vi "Update Library By Path.vi"(8 "error in":errorcluster, 9 "Library Path to be Replaced":path, 10 "Library":refnum<class "Library.lvclass">, 11 "Project in":refnum<class "Project.lvclass">) -> (0 "error out":errorcluster, 3 "Project out":refnum<class "Project.lvclass">)   [LabVIEW 2020, in "Panther Dashboard.lvlib" / "Project.lvclass"]
uses:
  Project.lvclass
  Library/Library.lvclass
  C:/GitClones/PantherDashboard/src/LabVIEW/Panther Dashboard/Class/LabVIEWItem/LabVIEWItem.lvclass
  Project.lvclass/Project.ctl
  LabVIEWItem/LabVIEWItem.lvclass/LabVIEWItem.ctl
  LabVIEWItem/Read Item Path.vi
  Read Libraries.vi
  Write Libraries.vi
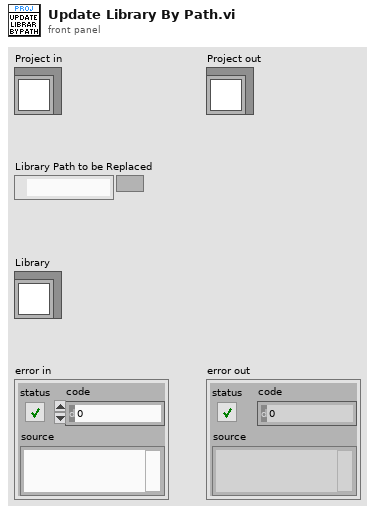
[diagram p1: front panel]
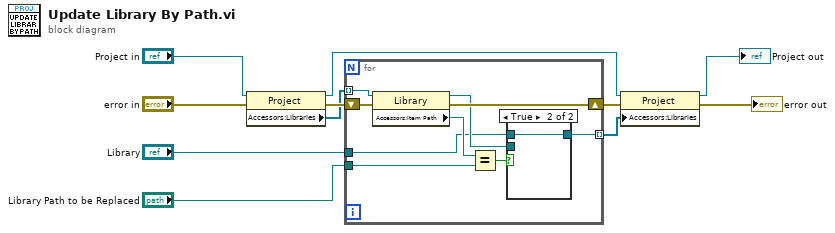
[diagram p0: block diagram]
diagram:
  n1 = property class="Project"(reference="Project in", error in="error in") -> (reference out=w5:refnum<class "Project.lvclass">, error out=w9:errorcluster, "Accessors:Libraries"=w2:refnum<class "Library.lvclass">[])
  n2 = for {
    tunnel: w2 -> [w18] mode=indexing
    tunnel: "Library" -> [w13]
    tunnel: "Library Path to be Replaced" -> [w16]
    tunnel: [w12] -> w6 mode=indexing
    shift-right: [w19] -> w8
    shift-left: w9 -> [w20]
    n3 = property class="Library"(reference=w18, error in=w20) -> (reference out=w14:refnum<class "Library.lvclass">, error out=w19:errorcluster, "Accessors:Item Path"=w17:path)
    n4 = Equal?(x=w17, y=w16) -> (x = y?=w15:bool)
    n5 = case shown="True" w15 {
      tunnel: w14 -> [w21 _]
      tunnel: w13 -> [_ w22]
      tunnel: [w21 w22] -> w12
      frame False {
      }
      frame True {
      }
    }
  }
  n6 = property class="Project"(reference=w5, error in=w8, "Accessors:Libraries"=w6) -> (reference out=→"Project out":refnum<class "Project.lvclass">, error out=→"error out":errorcluster)
